vi "7-OCU Dave.vi"() -> ()   [LabVIEW 2010]
doc: "This VI contrains the Forebrain within the Olin Robot Architecture. It must be run first to load the appropriate mission definition files. It contains a finite state machine built around a tabbed Operator interface that will guide an operator through the startup, run shutdown mission sequence. After running it, run the Midbrain and Hindbrain VIS."
uses:
  7-OCU/TabEnum.ctl
  4-High Neurons/MDFArray.ctl
  4-High Neurons/MissionDefinitionFile.ctl
  6-OCU Neurons/6.1-Act.ctl
  6-OCU Neurons/MainIndicators.ctl
  4-High Neurons/Current GPS Data.ctl
  3-Midbrain/3.2-Where/_typedefs/3.2.1-VectorNav Data.ctl
  4-High Neurons/4.2-Where Sensor Typedef.ctl
  3-Midbrain/3.3-What/_typedefs/3.3.1-LIDAR Data Typedef.ctl
  4-High Neurons/4.3-What Sensor Typedef.ctl
  6-OCU Neurons/6.4-How Reporting Typedef.ctl
  6-OCU Neurons/6.1-UDP Saitek.ctl
panel:
  out "ignore me 2":bool
  out "ignore me":bool
  in  "MissionDefinition":T1={"Waypoint #"=2.0, "X (waypoint)"=0.0, "Y (waypoint)"=0.0, "Vel (desired)"=0.0, "Dwell Time"=0.0, "Behavior"=enum."OpenFieldTransit", "Expand1"=0.0, "Expand2"=0.0, "Expand3"=0.0}
  out "(xr,yr) A":cluster{"X":dbl, "Y":dbl}
  out "What?Midbrain":cluster{"T":dbl, "Range":dbl, "Bearing":dbl}[](array[cluster])
  out "How?Midbrain":cluster{"T":dbl, "Battery":dbl, "Temp":dbl}
  out "What?Forebrain":cluster{"T":dbl, "Range":dbl, "Bearing":dbl}[](array[cluster])
  out "How?Forebrain":cluster{"T":dbl, "Battery":dbl, "Temp":dbl}
  out "Where? Forebrain":T2
  out "WhereAmI? Clean":T2
  out "(xr,yr)":cluster{"X":dbl, "Y":dbl}
  out "How?ForebrainOut":cluster{"T":dbl, "Battery":dbl, "Temp":dbl}
  out "How?MidbrainMM":cluster{"T":dbl, "Battery":dbl, "Temp":dbl}
  out "WhereAmI?MidB":T2
  out "Where?Forebrain":T2
  out "WhatAroundMe?MidB":cluster{"T":dbl, "Range":dbl, "Bearing":dbl}[](array[cluster])
  in  "RunRobot":bool
  out "Robot Live":bool
  in  "E-Stop":bool
  in  "Main Tab Interface":T3
  out "StartMissionMap":picture
  out "BatteryState":dbl(slide) scale=20.0..24.0
  out "LIDARCheck":picture
  out "MissionTime S&S":dbl(knob) scale=0.0..10.0
  out "CollisionWarning":bool
  out "DebugLIDAR":picture
  in  "SubPosition":T4 {"xrobot" min=0.0 max=300.0; "yrobot" min=0.0 max=300.0; "heading" min=-7.0 max=7.0 step=0.01}
  in  "LIDARControl":T5
  out "LIDAR Data (r:pixel b:degrees)":cluster{"Range":dbl, "Bearing":dbl}[](array[cluster])
  in  "Stop DebugSENSE":bool
  out "MissionMap":picture
  out "MDF Out":T6
  out "initialized MDF":T6
  in  "MDFile":T1
  out "Way Point Index":i32
  out "InitialWaypoint":cluster{"X":i16, "Y":i16}
  in  "Pen Color":u32(colorbox)=15671808
  in  "Select Pen Attributes":T7={"Width"=1, "Style"=enum."Solid"}
  out "Draw??":bool
  out "ManualActCommand":dbl[](array[numeric])
  out "Hypo Out":cluster{"Motor1":i16, "Motor 2":i16}
  out "NeoActCom":dbl[](array[numeric])
  out "SteerAngle":dbl
  in  "Load From File":bool
  in  "Save to File":bool
  out "MDF":T6
  in  "Select Your Behavior":T8(ring)
  out "No. of Waypoints":i32
  in  "Exit Planning":bool
  out "MissionDefFile":picture
  in  "RobotSpeed_Leg":dbl(slide) min=0.0 max=4.0 step=0.01 scale=0.0..4.0
  out "BuildMDF":bool
  out "ManualModeDatums":T9 {"5.3.1 MissionTimeAuto" scale=0.0..10.0; "4.2-Where Am I? Sensor"."4.2.2- Current GPS Data"."Longitude (dd.mmmmmm)" format="%#.6g"; "4.2-Where Am I? Sensor"."4.2.2- Current GPS Data"."Lattitude (dd.mmmmmm)" format="%#.6g"}
  in  "AutoModeDatums":T16 {"6.1-Saitek Controller"."Right" scale=-32767.0..32767.0; "6.1-Saitek Controller"."Left" scale=-32767.0..32767.0; "6.1-Saitek Controller"."Yaw" scale=-32767.0..32767.0; "6.1-Saitek Controller"."Roll" scale=-32767.0..32767.0; "6.1-Saitek Controller"."Pitch" scale=-32767.0..32767.0}
  out "Indicators":T9 {"5.3.1 MissionTimeAuto" scale=0.0..10.0; "4.2-Where Am I? Sensor"."4.2.2- Current GPS Data"."Longitude (dd.mmmmmm)" format="%#.6g"; "4.2-Where Am I? Sensor"."4.2.2- Current GPS Data"."Lattitude (dd.mmmmmm)" format="%#.6g"}
  out "Ready":bool
  out "CollisionLight 2":bool
  # "To run\nrobot,\nclick\narrow\nabove\n\nTo shut \noff \nrobot,\nclick \nbutton\nbelow."
  # "Operation Directions\n\n1)Click on Startup&\nShutdown tab.\n2) Click on Run \nArrow on menubar.\nRun Forebrain,\nMidbrain and Hindbrain.\n3) Select a mssion \nmap file when asked.\n4) Check robot is \nfully operational on\nStartup tab.\n5) Debug with debug\ntabs as required.\n6) Select ManualMode\ntab and test drive \nrobot.\n7) Select PlanMission\ntab and set up \nmission.\n8) Go to AutoMode\ntab and run mission."
  # "Turns off drive\nmotors"
  # "To operate:\n1) Run Forebrain.vi\n2) Run Midbrain.vi\n3) Run Hindbrain.vi"
  # "Use this tab\nto explore\nLIDAR\ndata and \noperation"
  # "Set \nX=130\nY=100\nto put\nrobot\nin center of\nMission\nMap"
  # "Set\nNumberOfBeams\nSensorRange\nNoise\nto\nview\nsimulated\nsensor\ndata"
  # "Directions:\n1) Select Robot Behavior for each mission leg.\n2) Select Robot Speed for leg.\n3) Select Robot Depth for leg.\n4) Click on robots current location for first waypoint.\n5) Click on next waypoint. Repeat for full mission.\n6) MDF will store up to 20 waypoints."
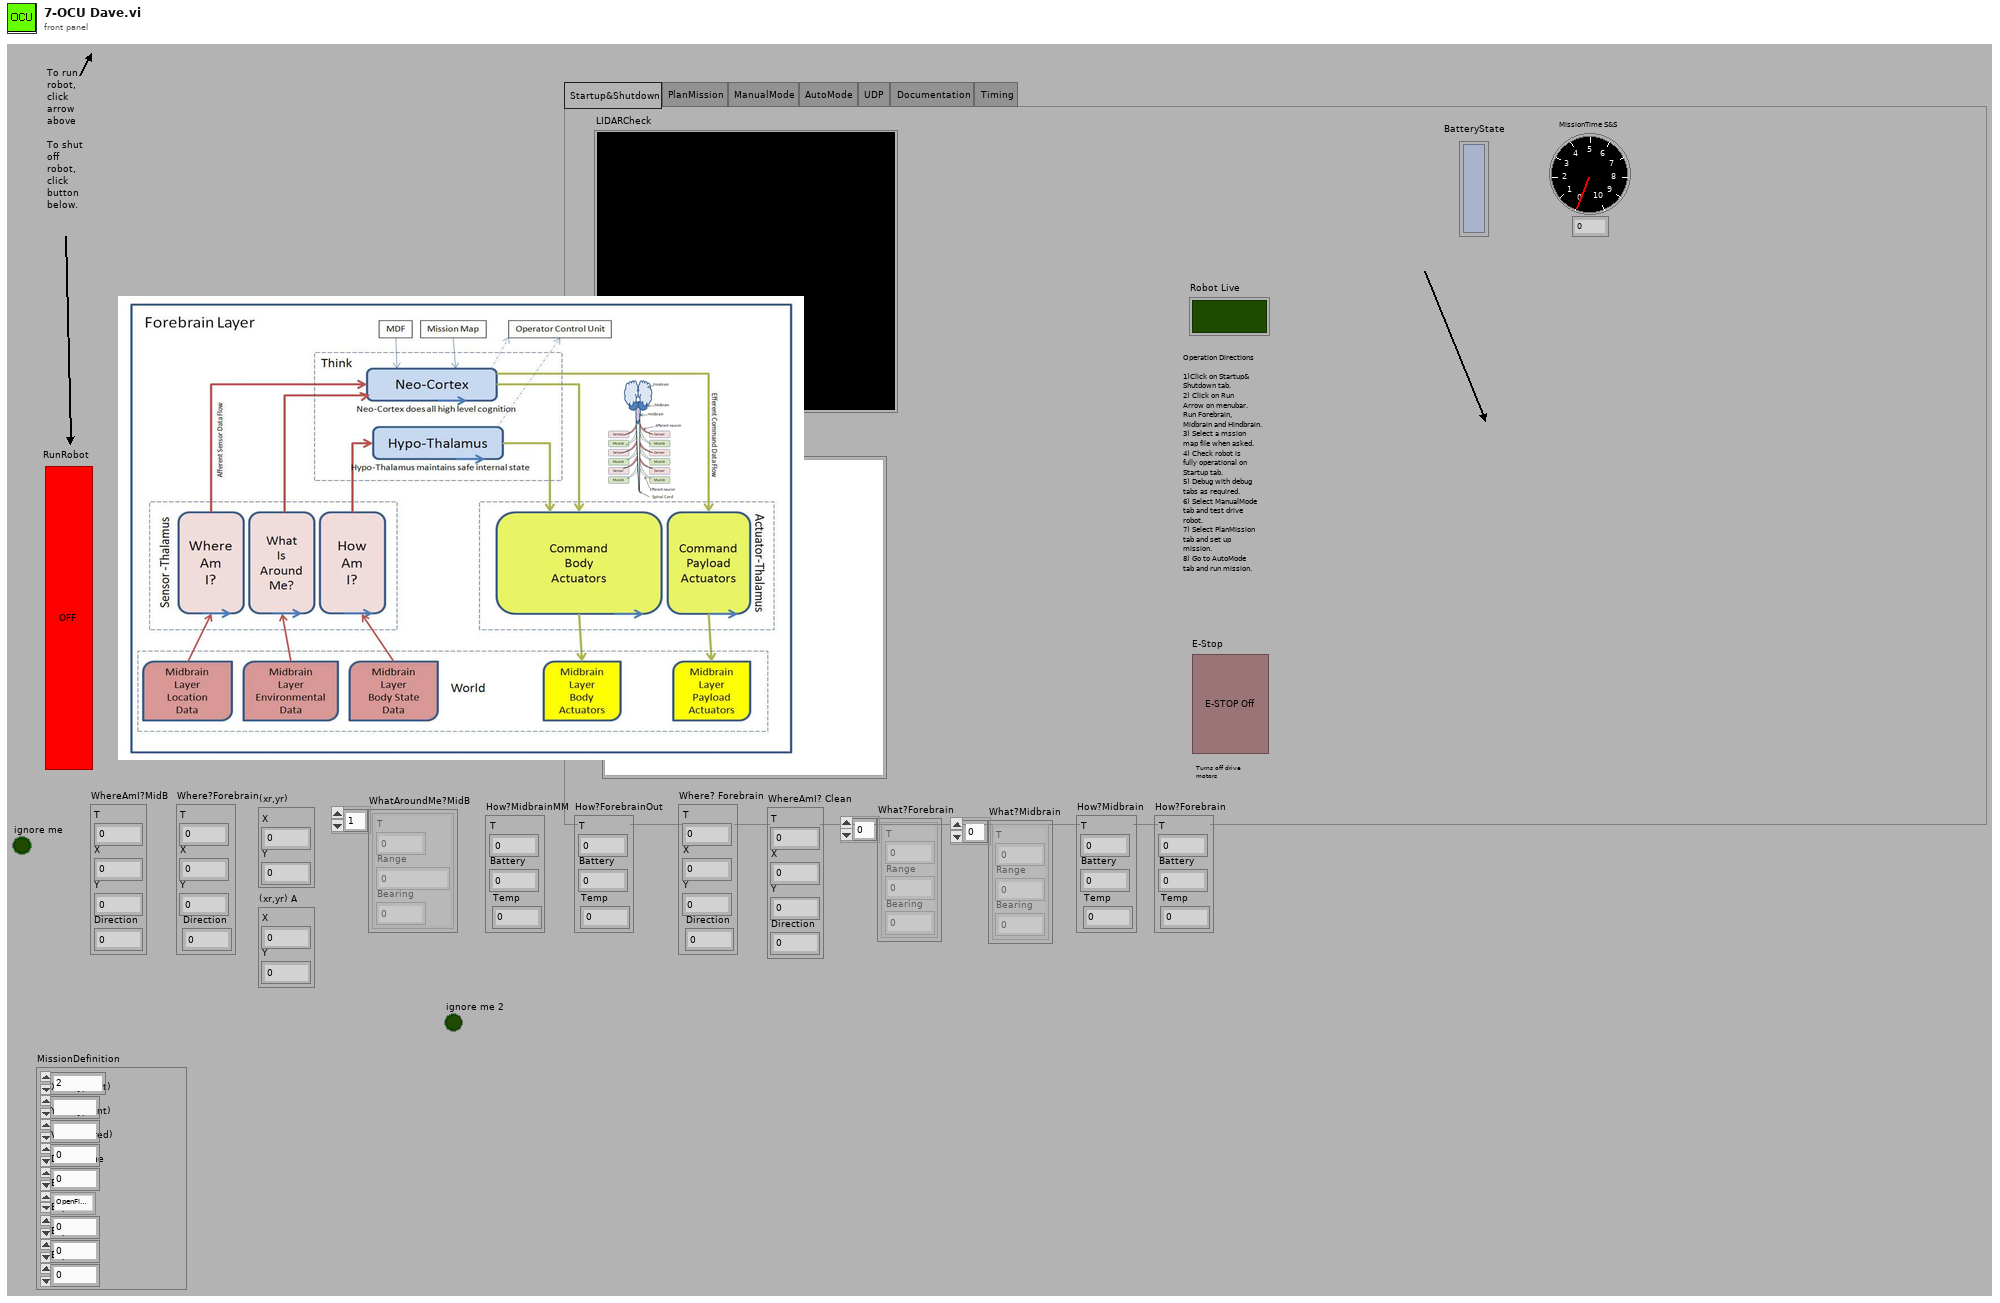
[diagram p1: front panel]
types:
  T1 = typedef "MissionDefinitionFile.ctl" = cluster{"Waypoint #":dbl, "X (waypoint)":ext, "Y (waypoint)":ext, "Vel (desired)":dbl, "Dwell Time":dbl, "Behavior":enum16{"OpenFieldTransit", "WallFollow", "LaneFollow", "ManualMode"}, "Expand1":dbl, "Expand2":dbl, "Expand3":dbl}
  T2 = cluster{"T":dbl, "X":dbl, "Y":dbl, "Direction":dbl}
  T3 = typedef "TabEnum.ctl" = enum32{"Startup&Shutdown", "PlanMission", "ManualMode", "AutoMode", "UDP", "Documentation", "Timing"}
  T4 = cluster{"xrobot":dbl, "yrobot":dbl, "heading":dbl}
  T5 = cluster{"NumberOfBeams":i32, "SensorRange":dbl, "Noise (0.1 to 1)":dbl}
  T6 = typedef "MDFArray.ctl" = T1[]
  T7 = cluster{"Width":u16, "Style":enum32{"Solid", "Dash", "Dot", "DashDot", "DashDotDot"}}
  T8 = enum16{"OpenFieldTransit", "WallFollow", "LaneFollow", "ManualMode"}
  T9 = typedef "MainIndicators.ctl" = cluster{"Where?":bool, "What?":bool, "4.2-Where Am I? Sensor":T10, "4.3-What's Around Me? Sensor":T13, "5.3.1 MissionTimeAuto":dbl, "5.4 Clean How Am I? Sensor":T15, "How?":bool}
  T10 = typedef "4.2-Where Sensor Typedef.ctl" = cluster{"4.2.2- Current GPS Data":T11, "4.2.1-VectorNav Data":T12, "4.2.1-VectorNav Status":string}
  T11 = typedef "Current GPS Data.ctl" = cluster{"Lattitude (dd.mmmmmm)":ext, "Longitude (dd.mmmmmm)":ext, "EST Time":timestamp}
  T12 = typedef "3.2.1-VectorNav Data.ctl" = cluster{"Yaw":dbl, "Pitch":dbl, "Roll":dbl}
  T13 = typedef "4.3-What Sensor Typedef.ctl" = cluster{"LIDAR Data":T14}
  T14 = typedef "3.3.1-LIDAR Data Typedef.ctl" = cluster{"Angle array":dbl[], "Magnitude array ":dbl[]}
  T15 = typedef "6.4-How Reporting Typedef.ctl" = cluster{"Motor Speed":i32, "Lidar Declination":i32, "Steering Angle":i32, "Battery Voltage":dbl, "Drive Encoder Cable Check":bool, "Lidar Drive Encoder Cable Check":bool, "Steer Encoder Cable Check":bool, "Lidar Pos Encoder Cable Check":bool, "Mod Buttons & Blinky Cable Check":bool, "Lidar Data Cable Check":bool, "Drive Motor Cable Check":bool, "Vector Nav Cable Check":bool, "Lidar Drive Cable Check":bool, "Steer Drive Cable Check":bool, "Reverse?":bool, "Steering Control Voltage":dbl, "Drive Control Voltage":dbl, "Lidar Control Voltage":dbl}
  T16 = typedef "6.1-Act.ctl" = cluster{"6.1-Saitek Controller":T17, "Manual Override":bool, "Shutdown":bool, "Reset":bool, "Begin":bool}
  T17 = typedef "6.1-UDP Saitek.ctl" = cluster{"Trig":bool, "2":bool, "3":bool, "4":bool, "5":bool, "6":bool, "7":bool, "8":bool, "9":bool, "10":bool, "11":bool, "Pitch":i32, "Ang":bool[], "Wheel":dbl, "Roll":i32, "Yaw":i32, "Left":i32, "Right":i32}
  T18 = enum32{"Startup&Shutdown", "DebugSENSE", "DebugTHINK", "DebugACT", "PlanMission", "ManualMode", "AutoMode", "Documentation"}
  T19 = cluster{"VelCom":dbl, "BehCom":enum16{"OpenFieldTransit", "WallFollow", "LaneFollow", "ManualMode"}}
  T20 = typedef "IMAQ Image.ctl" = refnum<image>
  T21 = typedef "imagedata.ctl" = cluster{"image type":i32, "image depth":i32, "image":u8[], "mask":u8[], "colors":u32[], "Rectangle":cluster{"left":i16, "top":i16, "right":i16, "bottom":i16}}
  T22 = typedef "LVMouseTypeDef.ctl" = cluster{"Mouse Position":cluster{"X":i32, "Y":i32}, "Mouse Modifiers":cluster{"Button Down":bool, "Shift Mod":bool, "Menu Mod":bool, "Option Mod":bool}}
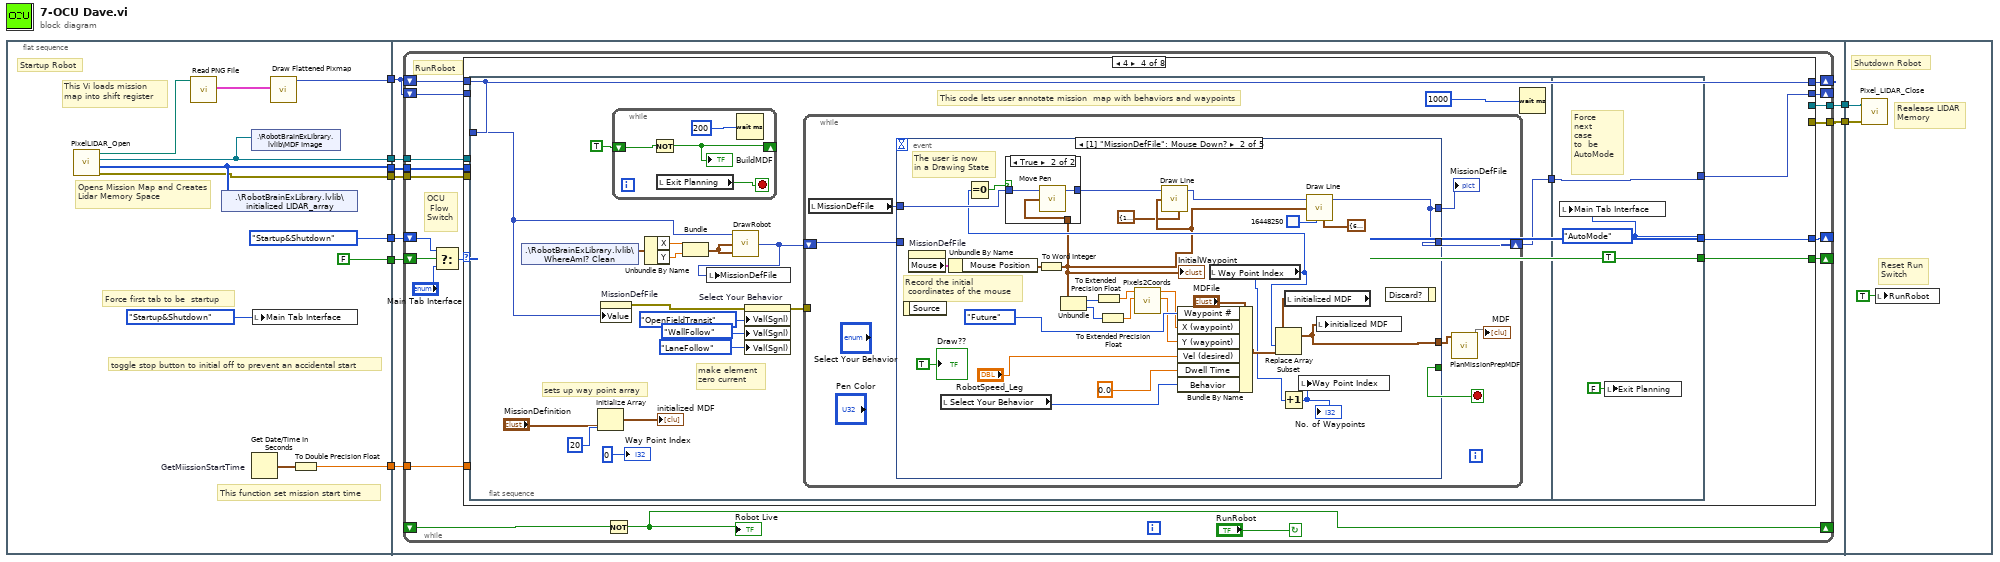
[diagram p0: block diagram]
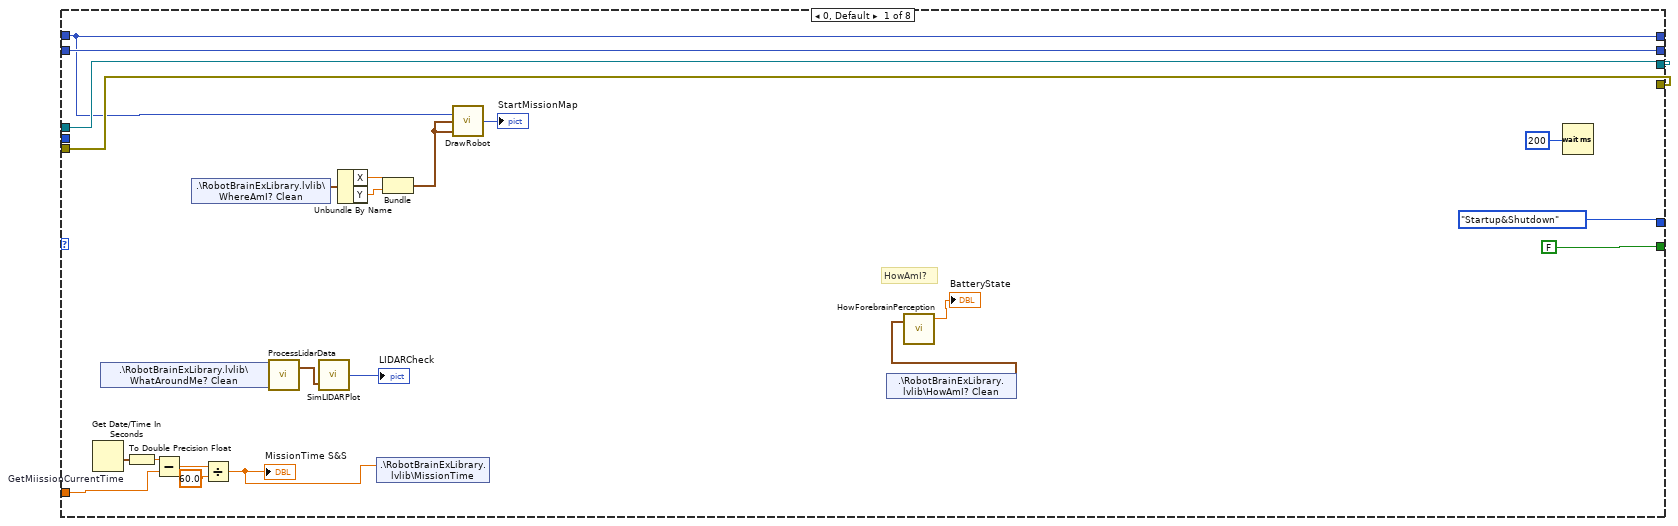
[diagram p2: hidden frame]
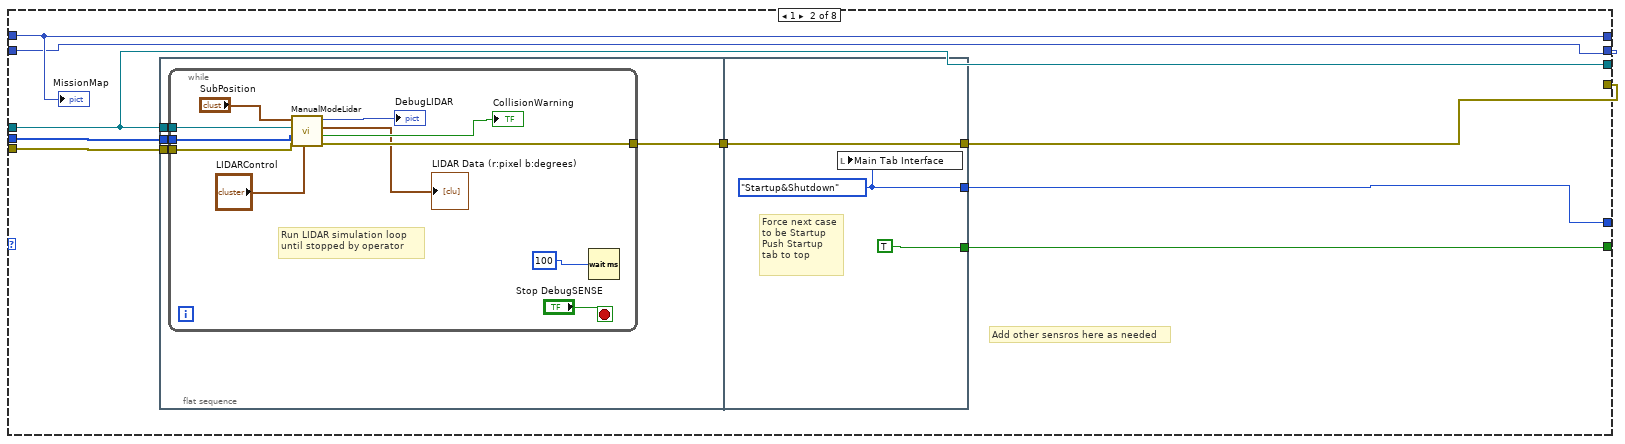
[diagram p3: hidden frame]
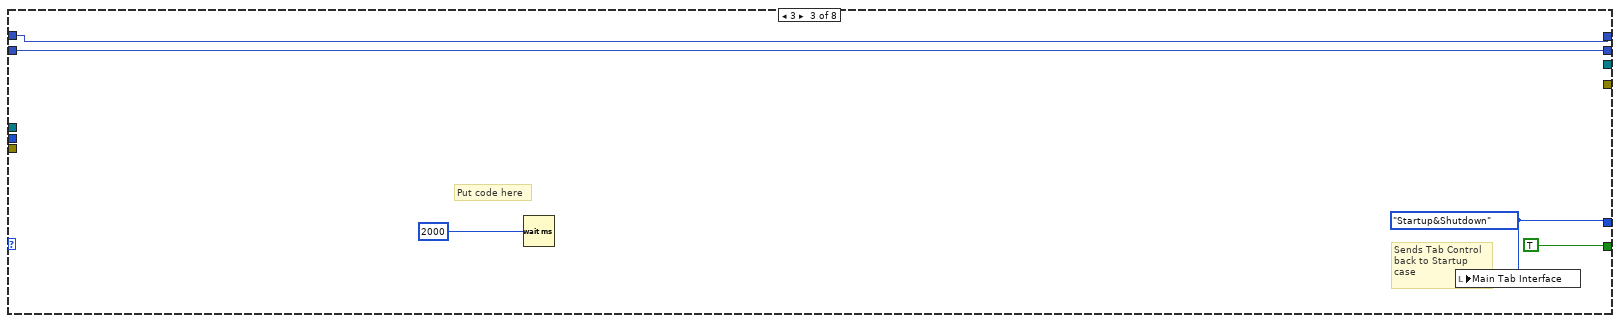
[diagram p4: hidden frame]
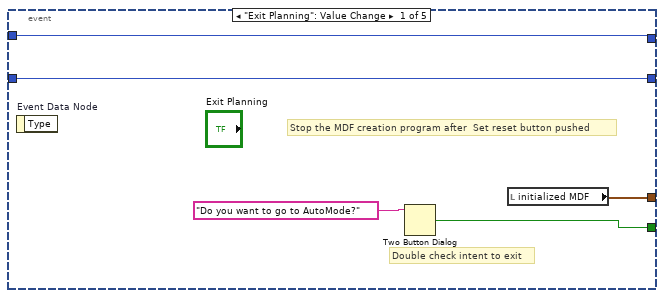
[diagram p5: hidden frame]
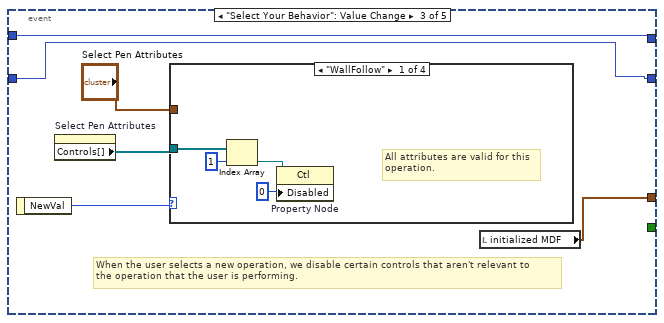
[diagram p7: hidden frame]
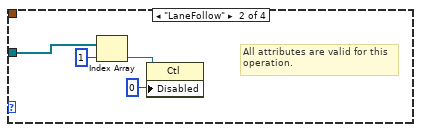
[diagram p8: hidden frame]
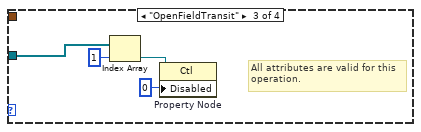
[diagram p9: hidden frame]
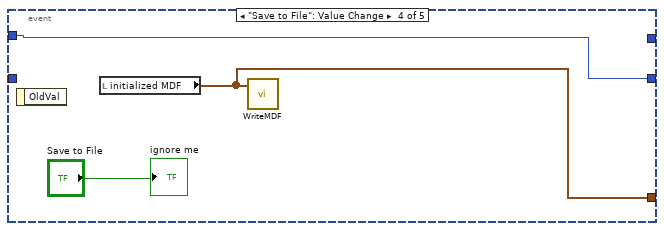
[diagram p11: hidden frame]
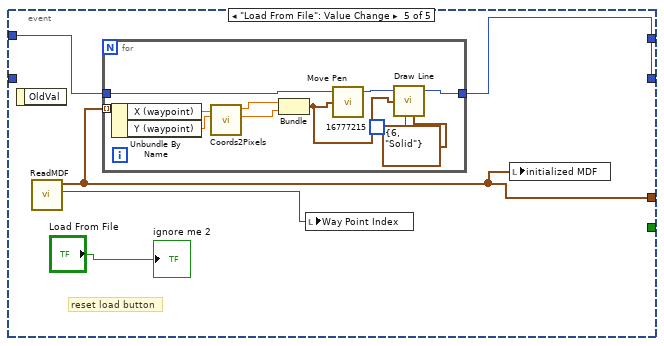
[diagram p12: hidden frame]
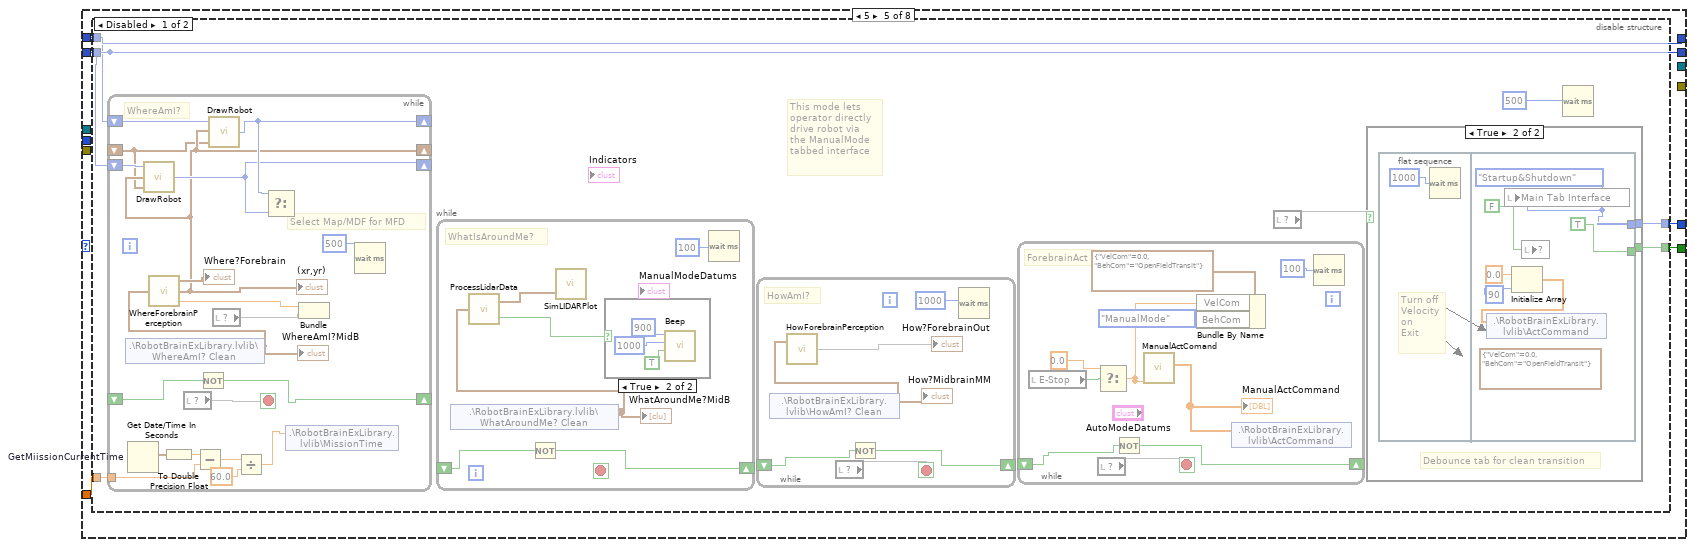
[diagram p13: hidden frame]
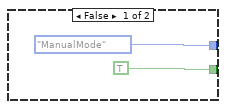
[diagram p15: hidden frame]
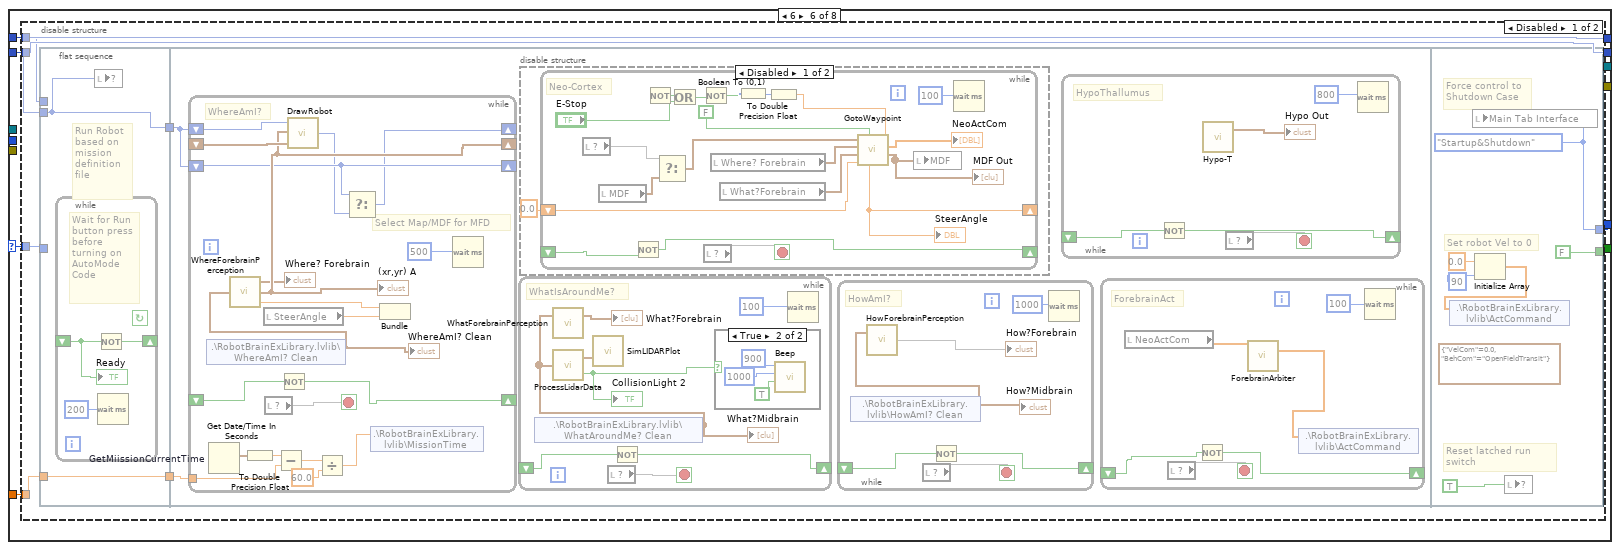
[diagram p17: hidden frame]
diagram:
  n1 = flat-sequence {
    tunnel: [w19] -> w9
    tunnel: [w17] -> w8
    tunnel: [w13] -> w7
    tunnel: [w15] -> w6
    tunnel: [w14] -> w5
    tunnel: [FALSE ("RunAutoMode")] -> w2
    tunnel: [T18."Startup&Shutdown" ("Tab")] -> w1
    tunnel: w9 -> [w29]
    tunnel: w8 -> [w28]
    tunnel: w7 -> [w27]
    tunnel: w6 -> [w26]
    tunnel: w5 -> [w25]
    tunnel: [w24] -> w4
    tunnel: [w23] -> w3
    tunnel: w2 -> [w22]
    tunnel: w1 -> [w21]
    tunnel: w4 -> [w405]
    tunnel: w3 -> [w404]
    frame #0 {
      # "Force first tab to be  startup"
      # "toggle stop button to initial off to prevent an accidental start"
      # "Opens Mission Map and Creates Lidar Memory Space"
      # "This function set mission start time"
      # "This Vi loads mission map into shift register"
      # "Startup Robot"
      n2 = call "PixelLIDAR_Open.vi"() -> ("error out"=w14:errorcluster, "initialized LIDAR\narray"=w15:i32[], "MDF Image"=w13:T20, "MissionMap"=w16:path)  [unwired: 2 in]
      n3 = call <vilib>:"Read PNG File.vi"("path to PNG file"=w16) -> ("image data"=w18:T21)  [unwired: 8 in, 2 out]
      n4 = shared-variable ".\\RobotBrainExLibrary.lvlib\\initialized LIDAR_array"(w15) -> ()  [unwired: 1 in, 1 out]
      n5 = shared-variable ".\\RobotBrainExLibrary.lvlib\\MDF Image"(w13) -> ()  [unwired: 1 in, 1 out]
      n6 = Get Date/Time In Seconds "GetMiissionStartTime"() -> (seconds since 1Jan1904=w20:timestamp)
      n7 = local write "Main Tab Interface"(T18."Startup&Shutdown" ("Tab")) -> ()
      n8 = call <vilib>:"Draw Flattened Pixmap.vi"("image data"=w18) -> ("new picture"=w17:picture)  [unwired: 8 in]
      n9 = To Double Precision Float(number=w20) -> (double precision float=w19:dbl)
    }
    frame #1 {
      n10 = while {
        shift-right: [w30] -> _
        shift-left: _ -> [w47]
        shift-right: [w46] -> _
        shift-left: w21 -> [w45]
        shift-right: [w42] -> _
        shift-left: w22 -> [w41]
        tunnel: w29 -> [w40]
        shift-right: [w38] -> _
        shift-left: w28 -> [w39]
        shift-right: [w36] -> _
        shift-left: w28 -> [w37]
        tunnel: w27 -> [w35]
        tunnel: w26 -> [w34]
        tunnel: w25 -> [w33]
        tunnel: [w32] -> w24
        tunnel: [w31] -> w23
        stop <- "RunRobot" continue-if-true
        # "RunRobot"
        # "OCU\n Flow\nSwitch"
        n11 = Select(t=w45, s=w41, f="Main Tab Interface") -> (s? t:f=w43:u32)
        n12 = case shown="4" w43 {
          selector: w43 -> [_ _ _ _ _ w296 _ _]
          tunnel: [T18."Startup&Shutdown" ("Tab") w75 w101 w108 w219 w297 T18."Startup&Shutdown" ("Tab") w402] -> w46
          tunnel: [FALSE ("s") w74 TRUE ("s") w107 w220 w295 FALSE ("s") TRUE ("s")] -> w42
          tunnel: w40 -> [w64 _ _ _ w218 w294 _ _]
          tunnel: w39 -> [w56 w77 w100 w104 w216 w292 w395 w400]
          tunnel: [w56 w77 w100 w104 w216 w292 w395 w400] -> w38
          tunnel: w37 -> [w63 w72 w99 _ w217 w293 w394 w399]
          tunnel: [w63 w72 w99 w105 w217 w293 w394 w399] -> w36
          tunnel: w35 -> [w62 w73 _ _ _ _ _ _]
          tunnel: w34 -> [_ w80 _ _ _ _ _ _]
          tunnel: w33 -> [w61 w79 _ _ _ _ _ _]
          tunnel: [w62 w73 _ _ _ _ _ _] -> w32
          tunnel: [w61 w78 _ _ _ _ _ _] -> w31
          frame 0, Default {
            # "HowAmI?"
            n13 = Get Date/Time In Seconds "GetMiissionCurrentTime"() -> (seconds since 1Jan1904=w68:timestamp)
            n14 = shared-variable ".\\RobotBrainExLibrary.lvlib\\WhatAroundMe? Clean"() -> (w57:cluster{"T":dbl, "Range":dbl, "Bearing":dbl}[])  [unwired: 1 in, 1 out]
            n15 = To Double Precision Float(number=w68) -> (double precision float=w67:dbl)
            n16 = Subtract(x=w67, y=w64) -> (x-y=w66:dbl)
            n17 = shared-variable ".\\RobotBrainExLibrary.lvlib\\WhereAmI? Clean"() -> (w52:T2)  [unwired: 1 in, 1 out]
            n18 = Divide(x=w66, y=60.0) -> (x/y=w60:dbl)
            "MissionTime S&S" <- w60
            n19 = call "ProcessLidarData.vi"("WhatAroundMe?MM"=w57) -> ("data array [mag, phase (deg)]"=w58:cluster{"magnitude":dbl, "phase":dbl}[])  [unwired: 1 out]
            n20 = call "SimLIDARPlot.vi"("data array [mag, phase (deg)]"=w58) -> ("SONAR"=→"LIDARCheck":picture)  [unwired: 1 in]
            n21 = Unbundle By Name(w52) -> ("X"=w51:dbl, "Y"=w50:dbl)
            n22 = shared-variable ".\\RobotBrainExLibrary.lvlib\\MissionTime"(w60) -> ()  [unwired: 1 in, 1 out]
            n23 = Bundle("X"=w51, "Y"=w50) -> (w49:cluster{"X":dbl, "Y":dbl})  [unwired: 1 in]
            n24 = call "DrawRobot.vi"("(xr,yr) old"=w49, "(xr,yr) new"=w49, "2D Picture"=w56) -> ("new picture"=→"StartMissionMap":picture)
            n25 = shared-variable ".\\RobotBrainExLibrary.lvlib\\HowAmI? Clean"() -> (w54:cluster{"T":dbl, "Battery":dbl, "Temp":dbl})  [unwired: 1 in, 1 out]
            n26 = call "HowForebrainPerception.vi"("How?MidbrainIn"=w54) -> ("BatteryGauge"=→"BatteryState":dbl)  [unwired: 3 in]
            n27 = Wait (ms)(milliseconds to wait=u32 200) -> ()  [unwired: 1 out]
          }
          frame 1 {
            # "Add other sensros here as needed"
            n28 = flat-sequence {
              tunnel: w80 -> [w84]
              tunnel: w79 -> [w83]
              tunnel: w73 -> [w82]
              tunnel: [w81] -> w76
              tunnel: [w98] -> w78
              tunnel: w76 -> [w98]
              tunnel: [w97] -> w75
              tunnel: [TRUE ("s")] -> w74
              frame #0 {
                n29 = while {
                  tunnel: w84 -> [w95]
                  tunnel: w83 -> [w94]
                  tunnel: w82 -> [w93]
                  tunnel: [w92] -> w81
                  stop <- "Stop DebugSENSE" stop-if-true
                  # "Run LIDAR simulation loop\nuntil stopped by operator"
                  n30 = call "ManualModeLidar.vi"("LIDARControl"="LIDARControl", "error in"=w94, "initialized \nsonar ray\narray"=w95, "MDF Image"=w93, "SubPosition"="SubPosition") -> ("error out"=w92:errorcluster, "Collision\nWarning"=→"CollisionWarning":bool, "LIDAR Data (r:pixel b:degrees)"=→"LIDAR Data (r:pixel b:degrees)":cluster{"Range":dbl, "Bearing":dbl}[], "LIDAR"=→"DebugLIDAR":picture)  [unwired: 1 in]
                  n31 = Wait (ms)(milliseconds to wait=u32 100) -> ()  [unwired: 1 out]
                }
              }
              frame #1 {
                w97 = T18."Startup&Shutdown" ("Tab")
                # "Force next case\nto be Startup\nPush Startup\ntab to top"
                n32 = local write "Main Tab Interface"(w97) -> ()
              }
            }
            "MissionMap" <- w77
          }
          frame 3 {
            w101 = T18."Startup&Shutdown" ("Tab")
            # "Put code here"
            # "Sends Tab Control\nback to Startup\ncase"
            n33 = Wait (ms)(milliseconds to wait=u32 2000) -> ()  [unwired: 1 out]
            n34 = local write "Main Tab Interface"(w101) -> ()
          }
          frame 4 {
            n35 = flat-sequence {
              tunnel: [w125] -> w106
              tunnel: w104 -> [w110]
              tunnel: [w214] -> w108
              tunnel: [TRUE ("s")] -> w107
              tunnel: w106 -> [w213]
              tunnel: [w213] -> w105
              frame #0 {
                # "make element \nzero current"
                # "sets up way point array"
                # "This code lets user annotate mission  map with behaviors and waypoints"
                n36 = shared-variable ".\\RobotBrainExLibrary.lvlib\\WhereAmI? Clean"() -> (w114:T2)  [unwired: 1 in, 1 out]
                n37 = Initialize Array ("Initialize WaypointArray")("MissionDefinition", 20 ("dimension size")) -> (→"initialized MDF":T1[])
                n38 = property on="MissionDefFile" class="Pict"("Value"=w110) -> (error out=w123:errorcluster)  [unwired: 2 in, 1 out]
                n39 = while {
                  shift-right: [w129] -> _
                  shift-left: TRUE -> [w130]
                  stop <- w128 stop-if-true
                  n40 = Not(x=w130) -> (.not. x?=w129:bool)
                  "BuildMDF" <- w129
                  n41 = local read "Exit Planning"() -> (w128:bool)
                  n42 = Wait (ms)(milliseconds to wait=u32 200) -> ()  [unwired: 1 out]
                }
                n43 = Unbundle By Name(w114) -> ("X"=w113:dbl, "Y"=w112:dbl)
                n44 = Bundle("X"=w113, "Y"=w112) -> (w111:cluster{"X":dbl, "Y":dbl})  [unwired: 1 in]
                n45 = call "DrawRobot.vi"("(xr,yr) old"=w111, "(xr,yr) new"=w111, "2D Picture"=w110) -> ("new picture"=w109:picture)
                n46 = local write "MissionDefFile"(w109) -> ()
                n47 = property on="Select Your Behavior" class="Enum (strict)"(error in=w123, "Val(Sgnl)"=T8."OpenFieldTransit" ("Select Your Behavior"), "Val(Sgnl)"=T8."WallFollow" ("Value (Signaling)"), "Val(Sgnl)"=T8."LaneFollow" ("Select Your Behavior")) -> (error out=w124:errorcluster)  [unwired: 1 in, 1 out]
                n48 = while {
                  shift-right: [w136] -> w125
                  shift-left: w109 -> [w137]
                  tunnel: w124 -> [_]
                  stop <- w135 stop-if-true
                  n49 = local read "MissionDefFile"() -> (w134:picture)
                  n50 = event shown="[1] \"MissionDefFile\": Mouse Down?" {
                    selector: _ -> [_ _ _ _ _]
                    dyn-events: _ -> [_ _ _ _ _]
                    timeout: _ -> [_ _ _ _ _]
                    tunnel: [w140 w153 w175 w194 w196] -> w136
                    tunnel: w137 -> [w140 _ w175 _ _]
                    tunnel: [w141 _ _ _ _] -> w135
                    tunnel: [w139 w167 w177 w195 w198] -> w131
                    tunnel: w134 -> [w138 w154 w176 w194 w197]
                    tunnel: [w138 w153 w176 _ _] -> w133
                    event "Exit Planning": Value Change {
                      # "Double check intent to exit"
                      # "Stop the MDF creation program after  Set reset button pushed"
                      n51 = event-data "Event Data Node"() -> ()  [unwired: 1 in, 1 out]
                      n52 = Two Button Dialog(message="Do you want to go to AutoMode?") -> (T button?=w141:bool)  [unwired: 2 in]
                      n53 = local read "initialized MDF"() -> (w139:T6)
                    }
                    event "MissionDefFile": Mouse Down? {
                      # "Record the initial\n coordinates of the mouse"
                      # "The user is now\nin a Drawing State"
                      n54 = event-data() -> ()  [unwired: 1 in, 1 out]
                      n55 = property on="MissionDefFile" class="Pict"() -> ("Mouse"=w170:T22)  [unwired: 2 in, 2 out]
                      n56 = local read "Select Your Behavior"() -> (w161:T8)
                      n57 = Unbundle By Name(w170) -> ("Mouse Position"=w168:cluster{"X":i32, "Y":i32})
                      n58 = To Word Integer(number=w168) -> (16bit integer=w144:cluster{"X":i16, "Y":i16})
                      "InitialWaypoint" <- w144
                      n59 = Unbundle(w144) -> ("X"=w163:i16, "Y"=w162:i16)
                      n60 = To Extended Precision Float(1:w163) -> (0:w151:ext)
                      n61 = To Extended Precision Float(1:w162) -> (0:w150:ext)
                      n62 = call "Pixels2Coords.vi"("Y (pixels)"=w150, "X (pixels)"=w151) -> ("Latitude"=w148:ext, "Longtitude"=w149:ext)  [unwired: 8 in]
                      n63 = Bundle By Name(cluster="MDFile", "Waypoint #"=enum16{"Past", "Current", "Future"}."Future" ("Status"), "X (waypoint)"=w149, "Y (waypoint)"=w148, "Vel (desired)"="RobotSpeed_Leg", "Dwell Time"=0.0, "Behavior"=w161) -> (w164:T1)
                      n64 = local read "Way Point Index"() -> (w147:i32)
                      n65 = Equal To 0?(x=w147) -> (x = 0?=w146:bool)
                      n66 = case shown="True" w146 {
                        tunnel: [w171 w174] -> w157
                        tunnel: w144 -> [_ w173]
                        tunnel: w154 -> [w171 w172]
                        frame False {
                        }
                        frame True {
                          n67 = call <vilib>:"Move Pen.vi"("new position"=w173, "picture"=w172) -> ("new picture"=w174:picture)  [unwired: 3 in]
                        }
                      }
                      n68 = call <vilib>:"Draw Line.vi"("picture"=w157, "end point"=w144, "pen"=T7 {"Width"=1, "Style"=enum."Dot"}) -> ("new picture"=w145:picture)  [unwired: 6 in]
                      n69 = Increment(x=w147) -> (x+1=w169:i32)
                      "No. of Waypoints" <- w169
                      n70 = local read "initialized MDF"() -> (w166:T6)
                      n71 = Replace Array Subset(array=w166, new element=w164, index=w147) -> (w167:T6)
                      n72 = local write "Way Point Index"(w169) -> ()
                      n73 = call <vilib>:"Draw Line.vi"("picture"=w145, "end point"=w144, "color(black)"=u32 16448250, "pen"=T7 {"Width"=6, "Style"=enum."Solid"}) -> ("new picture"=w153:picture)  [unwired: 5 in]
                      n74 = local write "initialized MDF"(w167) -> ()
                      n75 = event-data() -> ()  [unwired: 2 in, 1 out]
                      "Draw??" <- TRUE ("Draw??")
                    }
                    event "Select Your Behavior": Value Change {
                      # "When the user selects a new operation, we disable certain controls that aren't relevant to\nthe operation that the user is performing."
                      n76 = event-data() -> ("NewVal"=w180:T8)  [unwired: 1 in]
                      n77 = property on="Select Pen Attributes" class="Clust (strict)"() -> ("Controls[]"=w179:refnum<vi>[])  [unwired: 2 in, 2 out]
                      n78 = case shown="\"WallFollow\"" w180 {
                        tunnel: w179 -> [w184 w185 w189 _]
                        tunnel: "Select Pen Attributes" -> [_ _ _ _]
                        frame "WallFollow" {
                          # "All attributes are valid for this\noperation."
                          n79 = Index Array "Index Array"(array=w184, index=1) -> (element=w182:refnum<vi>)
                          n80 = property on="Property Node" class="Ctl"(reference=w182, "Disabled"=u8 0) -> ()  [unwired: 1 in, 2 out]
                        }
                        frame "LaneFollow" {
                          # "All attributes are valid for this\noperation."
                          n81 = Index Array(array=w185, index=1) -> (element=w187:refnum<vi>)
                          n82 = property class="Ctl"(reference=w187, "Disabled"=u8 0) -> ()  [unwired: 1 in, 2 out]
                        }
                        frame "OpenFieldTransit" {
                          # "All attributes are valid for this\noperation."
                          n83 = Index Array "Index Array"(array=w189, index=1) -> (element=w191:refnum<vi>)
                          n84 = property on="Property Node" class="Ctl"(reference=w191, "Disabled"=u8 0) -> ()  [unwired: 1 in, 2 out]
                        }
                        frame "ManualMode" {
                        }
                      }
                      n85 = local read "initialized MDF"() -> (w177:T6)
                    }
                    event "Save to File": Value Change {
                      n86 = event-data() -> ()  [unwired: 1 in, 1 out]
                      n87 = local read "initialized MDF"() -> (w195:T6)
                      n88 = call "WriteMDF.vi"(11:w195) -> ()  [unwired: 11 in]
                      "ignore me" <- "Save to File"
                    }
                    event "Load From File": Value Change {
                      # "reset load button"
                      n89 = event-data() -> ()  [unwired: 1 in, 1 out]
                      n90 = call "ReadMDF.vi"() -> ("Number of Waypoints Read"=w199:i32, "MDF Array out"=w198:T6)  [unwired: 10 in]
                      n91 = for {
                        tunnel: w198 -> [w211] mode=indexing
                        tunnel: w197 -> [w210]
                        tunnel: [w208] -> w196
                        n92 = Unbundle By Name(w211) -> ("X (waypoint)"=w204:ext, "Y (waypoint)"=w203:ext)
                        n93 = call "Coords2Pixels.vi"("Latitude"=w203, "Longitude"=w204) -> ("Y"=w201:ext, "X"=w202:ext)  [unwired: 8 in]
                        n94 = Bundle("X"=w202, "Y"=w201) -> (w207:cluster{"X":ext, "Y":ext})  [unwired: 1 in]
                        n95 = call <vilib>:"Move Pen.vi"("new position"=w207, "picture"=w210) -> ("new picture"=w209:picture)  [unwired: 3 in]
                        n96 = call <vilib>:"Draw Line.vi"("picture"=w209, "end point"=w207, "color(black)"=u32 16777215, "pen"=T7 {"Width"=6, "Style"=enum."Solid"}) -> ("new picture"=w208:picture)  [unwired: 5 in]
                      }
                      n97 = local write "Way Point Index"(w199) -> ()
                      n98 = local write "initialized MDF"(w198) -> ()
                      "ignore me 2" <- "Load From File"
                    }
                  }
                  "MissionDefFile" <- w133
                  n99 = call "PlanMissionPrepMDF.vi"(11:w131) -> (3:→"MDF")  [unwired: 9 in, 1 out]
                }
                n100 = Wait (ms)(milliseconds to wait=u32 1000) -> ()  [unwired: 1 out]
                "Way Point Index" <- 0 ("Boundary Point Index")
              }
              frame #1 {
                w214 = T18."AutoMode" ("Tab")
                # "Force \nnext \ncase\nto  be\nAutoMode"
                n101 = local write "Main Tab Interface"(w214) -> ()
                n102 = local write "Exit Planning"(FALSE ("Exit Planning")) -> ()
              }
            }
          }
          frame 5 {
            n103 = disable-structure shown="Disabled" {
              disable-tunnel: [w226 _] -> w220
              disable-tunnel: [w225 _] -> w219
              disable-tunnel: w218 -> [w223 _]
              disable-tunnel: w217 -> [w222 _]
              disable-tunnel: w216 -> [w221 _]
              frame Disabled {
                # "This mode lets \noperator directly\ndrive robot via\nthe ManualMode\ntabbed interface"
                n104 = while {
                  shift-right: [w250] -> _
                  shift-left: _ -> [w249]
                  tunnel: w223 -> [w242]
                  shift-right: [w232] -> _
                  shift-left: w221 -> [w235]
                  shift-right: [w229] -> _
                  shift-left: _ -> [w228]
                  shift-right: [w230] -> _
                  shift-left: w222 -> [w231]
                  stop <- w248 stop-if-true
                  # "Select Map/MDF for MFD"
                  # "WhereAmI?"
                  n105 = shared-variable ".\\RobotBrainExLibrary.lvlib\\WhereAmI? Clean"() -> (w241:T2)  [unwired: 1 in, 1 out]
                  "WhereAmI?MidB" <- w241
                  n106 = Get Date/Time In Seconds "GetMiissionCurrentTime"() -> (seconds since 1Jan1904=w243:timestamp)
                  n107 = call "WhereForebrainPerception.vi"("Where? Midbrain"=w241) -> ("SimPitchRoll"=w240:dbl, "Where? Forebrain"=→"Where?Forebrain":T2, "(xr,yr)"=w229:cluster{"X":dbl, "Y":dbl}, "Direction"=w239:dbl)  [unwired: 3 in]
                  "(xr,yr)" <- w229
                  n108 = call "DrawRobot.vi"("(xr,yr) old"=w228, "(xr,yr) new"=w229, "2D Picture"=w231) -> ("new picture"=w230:picture)
                  n109 = To Double Precision Float(number=w243) -> (double precision float=w244:dbl)
                  n110 = local read item#-1() -> (w248)
                  n111 = Subtract(x=w244, y=w242) -> (x-y=w245:dbl)
                  n112 = Not(x=w249) -> (.not. x?=w250:bool)
                  n113 = call "DrawRobot.vi"("(xr,yr) old"=w228, "(xr,yr) new"=w229, "2D Picture"=w235) -> ("new picture"=w232:picture)
                  n114 = local read item#-1() -> (w237)
                  n115 = Divide(x=w245, y=60.0) -> (x/y=w247:dbl)
                  n116 = Select(t=w232, f=w230) -> (s=w233:bool, s? t:f=w234:picture)
                  n117 = shared-variable ".\\RobotBrainExLibrary.lvlib\\MissionTime"(w247) -> ()  [unwired: 1 in, 1 out]
                  n118 = Bundle("Direction"=w239, w237) -> (w238:cluster{"Direction":dbl, void})  [unwired: 1 in]
                  n119 = Wait (ms)(milliseconds to wait=u32 500) -> ()  [unwired: 1 out]
                }
                n120 = while {
                  shift-right: [w257] -> _
                  shift-left: _ -> [w258]
                  stop <- w256 stop-if-true
                  # "WhatIsAroundMe?"
                  n121 = shared-variable ".\\RobotBrainExLibrary.lvlib\\WhatAroundMe? Clean"() -> (w253:cluster{"T":dbl, "Range":dbl, "Bearing":dbl}[])  [unwired: 1 in, 1 out]
                  "WhatAroundMe?MidB" <- w253
                  n122 = call "ProcessLidarData.vi"("WhatAroundMe?MM"=w253) -> ("Collision"=w252:bool, "data array [mag, phase (deg)]"=w254:cluster{"magnitude":dbl, "phase":dbl}[])
                  n123 = Not(x=w258) -> (.not. x?=w257:bool)
                  n124 = call "SimLIDARPlot.vi"("data array [mag, phase (deg)]"=w254) -> ("SONAR"=w255:picture)  [unwired: 1 in]
                  n125 = case shown="True" w252 {
                    frame False {
                      # "No \nBeep"
                    }
                    frame True {
                      n126 = call <vilib>:"Beep.vi"("use system alert? (T)"=TRUE, "duration (msec)"=u32 1000, "frequency (Hz)"=u32 900) -> ()  [unwired: 9 in]
                    }
                  }
                  n127 = Wait (ms)(milliseconds to wait=u32 100) -> ()  [unwired: 1 out]
                }
                n128 = while {
                  shift-right: [w279] -> _
                  shift-left: _ -> [w278]
                  stop <- w275 stop-if-true
                  # "HowAmI?"
                  n129 = shared-variable ".\\RobotBrainExLibrary.lvlib\\HowAmI? Clean"() -> (w277:cluster{"T":dbl, "Battery":dbl, "Temp":dbl})  [unwired: 1 in, 1 out]
                  "How?MidbrainMM" <- w277
                  n130 = call "HowForebrainPerception.vi"("How?MidbrainIn"=w277) -> (3:→"How?ForebrainOut")  [unwired: 2 in, 1 out]
                  n131 = local read item#-1() -> (w275)
                  n132 = Not(x=w278) -> (.not. x?=w279:bool)
                  n133 = Wait (ms)(milliseconds to wait=u32 1000) -> ()  [unwired: 1 out]
                }
                n134 = while {
                  shift-right: [w273] -> _
                  shift-left: _ -> [w272]
                  stop <- w270 stop-if-true
                  # "ForebrainAct"
                  n135 = local read "E-Stop"() -> (w264:bool)
                  n136 = Select(t=0.0, s=w264) -> (f=w265:dbl, s? t:f=w266:dbl)
                  n137 = local read item#-1() -> (w270)
                  n138 = Not(x=w272) -> (.not. x?=w273:bool)
                  n139 = call "ManualActComand.vi"("Speed"=w266) -> ("ManualActCommand"=w271:dbl[], "SteeringAngle"=w269:dbl)  [unwired: 9 in]
                  "ManualActCommand" <- w271
                  n140 = Bundle By Name(cluster=T19 {"VelCom"=0.0, "BehCom"=enum."OpenFieldTransit"} ("ForebrainCom"), "VelCom"=w266, "BehCom"=T8."ManualMode") -> ()  [unwired: 1 out]
                  n141 = shared-variable ".\\RobotBrainExLibrary.lvlib\\ActCommand"(w271) -> ()  [unwired: 1 in, 1 out]
                  n142 = Wait (ms)(milliseconds to wait=u32 100) -> ()  [unwired: 1 out]
                }
                n143 = local read item#-1() -> (w224)
                n144 = case shown="True" w224 {
                  tunnel: [TRUE ("s") w283] -> w226
                  tunnel: [T18."ManualMode" ("Tab") w284] -> w225
                  frame False {
                  }
                  frame True {
                    # "Debounce tab for clean transition"
                    n145 = flat-sequence {
                      tunnel: [w290] -> w284
                      tunnel: [TRUE ("s")] -> w283
                      frame #0 {
                        # "Turn off\nVelocity\non \nExit"
                        n146 = Wait (ms)(milliseconds to wait=u32 1000) -> ()  [unwired: 1 out]
                      }
                      frame #1 {
                        (unwired) T19 {"VelCom"=0.0, "BehCom"=enum."OpenFieldTransit"} ("ForebrainCom")
                        w290 = T18."Startup&Shutdown" ("Tab")
                        n147 = local write "Main Tab Interface"(w290) -> ()
                        n148 = Initialize Array(0.0 ("element"), 90 ("dimension size")) -> (w288:dbl[])
                        n149 = shared-variable ".\\RobotBrainExLibrary.lvlib\\ActCommand"(w288) -> ()  [unwired: 1 in, 1 out]
                        n150 = local write item#-1(FALSE ("ManualModeStop")) -> ()
                      }
                    }
                  }
                }
                n151 = Wait (ms)(milliseconds to wait=u32 500) -> ()  [unwired: 1 out]
              }
              frame Enabled {
              }
            }
          }
          frame 6 {
            n152 = disable-structure shown="Disabled" {
              disable-tunnel: [w303 _] -> w297
              disable-tunnel: w296 -> [w302 _]
              disable-tunnel: [w301 _] -> w295
              disable-tunnel: w294 -> [w300 _]
              disable-tunnel: w293 -> [w299 _]
              disable-tunnel: w292 -> [w298 _]
              frame Disabled {
                n153 = flat-sequence {
                  tunnel: w302 -> [_]
                  tunnel: [w307] -> w305
                  tunnel: w300 -> [w307]
                  tunnel: w299 -> [w306]
                  tunnel: [w306] -> w304
                  tunnel: w298 -> [_]
                  tunnel: w305 -> [w312]
                  tunnel: w304 -> [w311]
                  tunnel: [w392] -> w303
                  tunnel: [FALSE ("s")] -> w301
                  frame #0 {
                    # "Run Robot\nbased on\nmission\ndefinition\nfile"
                    n154 = while {
                      shift-right: [w310] -> _
                      shift-left: _ -> [w309]
                      stop <- _ continue-if-true
                      # "Wait for Run\nbutton press\nbefore\nturning on\nAutoMode\nCode"
                      n155 = Not(x=w309) -> (.not. x?=w310:bool)
                      n156 = Wait (ms)(milliseconds to wait=u32 200) -> ()  [unwired: 1 out]
                      "Ready" <- w309
                    }
                    n157 = local write item#-1(w306) -> ()
                  }
                  frame #1 {
                    n158 = while {
                      shift-right: [w386] -> _
                      shift-left: _ -> [w373]
                      tunnel: w312 -> [w381]
                      shift-right: [w365] -> _
                      shift-left: w311 -> [w368]
                      shift-right: [w378] -> _
                      shift-left: _ -> [w379]
                      shift-right: [w367] -> _
                      shift-left: w311 -> [w367]
                      stop <- w372 stop-if-true
                      # "Select Map/MDF for MFD"
                      # "WhereAmI?"
                      n159 = shared-variable ".\\RobotBrainExLibrary.lvlib\\WhereAmI? Clean"() -> (w375:T2)  [unwired: 1 in, 1 out]
                      "WhereAmI? Clean" <- w375
                      n160 = Get Date/Time In Seconds "GetMiissionCurrentTime"() -> (seconds since 1Jan1904=w382:timestamp)
                      n161 = call "WhereForebrainPerception.vi"("Where? Midbrain"=w375) -> ("SimPitchRoll"=w370:dbl, "Where? Forebrain"=→"Where? Forebrain":T2, "(xr,yr)"=w378:cluster{"X":dbl, "Y":dbl}, "Direction"=w380:dbl)  [unwired: 3 in]
                      "(xr,yr) A" <- w378
                      n162 = To Double Precision Float(number=w382) -> (double precision float=w383:dbl)
                      n163 = local read "SteerAngle"() -> (w369:dbl)
                      n164 = local read item#-1() -> (w372)
                      n165 = Subtract(x=w383, y=w381) -> (x-y=w384:dbl)
                      n166 = Not(x=w373) -> (.not. x?=w386:bool)
                      n167 = call "DrawRobot.vi"("(xr,yr) old"=w379, "(xr,yr) new"=w378, "2D Picture"=w368) -> ("new picture"=w366:picture)
                      n168 = Divide(x=w384, y=60.0) -> (x/y=w374:dbl)
                      n169 = Select(t=w367, f=w366) -> (s=w377:bool, s? t:f=w365:picture)
                      n170 = shared-variable ".\\RobotBrainExLibrary.lvlib\\MissionTime"(w374) -> ()  [unwired: 1 in, 1 out]
                      n171 = Bundle("Direction"=w380, "SteerAngle"=w369) -> (w371:cluster{"Direction":dbl, "SteerAngle":dbl})  [unwired: 1 in]
                      n172 = Wait (ms)(milliseconds to wait=u32 500) -> ()  [unwired: 1 out]
                    }
                    n173 = while {
                      shift-right: [w358] -> _
                      shift-left: _ -> [w360]
                      stop <- w357 stop-if-true
                      # "WhatIsAroundMe?"
                      n174 = shared-variable ".\\RobotBrainExLibrary.lvlib\\WhatAroundMe? Clean"() -> (w355:cluster{"T":dbl, "Range":dbl, "Bearing":dbl}[])  [unwired: 1 in, 1 out]
                      "What?Midbrain" <- w355
                      n175 = call "WhatForebrainPerception.vi"("What?Midbrain"=w355) -> ("What?Midbrain 2"=→"What?Forebrain":cluster{"T":dbl, "Range":dbl, "Bearing":dbl}[])  [unwired: 2 in]
                      n176 = call "ProcessLidarData.vi"("WhatAroundMe?MM"=w355) -> ("Collision"=w354:bool, "data array [mag, phase (deg)]"=w359:cluster{"magnitude":dbl, "phase":dbl}[])
                      "CollisionLight 2" <- w354
                      n177 = call "SimLIDARPlot.vi"("data array [mag, phase (deg)]"=w359) -> ()  [unwired: 1 in, 1 out]
                      n178 = local read item#-1() -> (w357)
                      n179 = Not(x=w360) -> (.not. x?=w358:bool)
                      n180 = case shown="True" w354 {
                        frame False {
                          # "No \nBeep"
                        }
                        frame True {
                          n181 = call <vilib>:"Beep.vi"("use system alert? (T)"=TRUE, "duration (msec)"=u32 1000, "frequency (Hz)"=u32 900) -> ()  [unwired: 9 in]
                        }
                      }
                      n182 = Wait (ms)(milliseconds to wait=u32 100) -> ()  [unwired: 1 out]
                    }
                    n183 = disable-structure shown="Disabled" {
                      frame Disabled {
                        n184 = while {
                          shift-right: [w333] -> _
                          shift-left: _ -> [w332]
                          shift-right: [w325] -> _
                          shift-left: 0.0 ("SteerAngle") -> [w324]
                          stop <- w335 stop-if-true
                          # "Neo-Cortex"
                          n185 = local read item#-1() -> (w317)
                          n186 = local read "MDF"() -> (w316:T6)
                          n187 = Not(x=w332) -> (.not. x?=w333:bool)
                          n188 = Not() -> (.not. x?=w321:bool)  [unwired: 1 in]
                          n189 = Select(t=w317, f=w316) -> (s=w315:bool, s? t:f=w314:T6)
                          n190 = Or(x=w321, y="E-Stop") -> (x .or. y?=w319:bool)
                          n191 = Not(x=w319) -> (.not. x?=w318:bool)
                          n192 = local read item#-1() -> (w335)
                          n193 = local read "Where? Forebrain"() -> (w331:T2)
                          n194 = local read "What?Forebrain"() -> (w330:cluster{"T":dbl, "Range":dbl, "Bearing":dbl}[])
                          n195 = Boolean To (0,1)(Boolean=w318) -> (0, 1=w323:i16)
                          n196 = To Double Precision Float(number=w323) -> (double precision float=w322:dbl)
                          n197 = call "GotoWaypoint.vi"("SupressIn"=w322, "InhibitIn"=FALSE, "CurrentSteerAngle"=w324, "WhatAroundMe? Clean"=w330, "WhereAmI? Clean"=w331, "MDF In"=w314) -> ("MDF Out"=w327:T6, "ActCommand"=→"NeoActCom":dbl[], "Vel"=w326:dbl, "SteerAngle"=w325:dbl)  [unwired: 2 out]
                          "SteerAngle" <- w325
                          "MDF Out" <- w327
                          n198 = local write "MDF"(w327) -> ()
                          n199 = Wait (ms)(milliseconds to wait=u32 100) -> ()  [unwired: 1 out]
                        }
                      }
                      frame Enabled {
                      }
                    }
                    n200 = while {
                      shift-right: [w352] -> _
                      shift-left: _ -> [w348]
                      stop <- w347 stop-if-true
                      # "HowAmI?"
                      n201 = shared-variable ".\\RobotBrainExLibrary.lvlib\\HowAmI? Clean"() -> (w349:cluster{"T":dbl, "Battery":dbl, "Temp":dbl})  [unwired: 1 in, 1 out]
                      "How?Midbrain" <- w349
                      n202 = call "HowForebrainPerception.vi"("How?MidbrainIn"=w349) -> (2:w350, 3:→"How?Forebrain")  [unwired: 1 in, 1 out]
                      n203 = local read item#-1() -> (w347)
                      n204 = Not(x=w348) -> (.not. x?=w352:bool)
                      n205 = Wait (ms)(milliseconds to wait=u32 1000) -> ()  [unwired: 1 out]
                    }
                    n206 = while {
                      shift-right: [w337] -> _
                      shift-left: _ -> [w338]
                      stop <- w340 stop-if-true
                      # "HypoThallumus"
                      n207 = Not(x=w338) -> (.not. x?=w337:bool)
                      n208 = call "Hypo-T.vi"() -> ("Hypo T Act Out"=→"Hypo Out":cluster{"Motor1":i16, "Motor 2":i16})  [unwired: 3 in]
                      n209 = local read item#-1() -> (w340)
                      n210 = Wait (ms)(milliseconds to wait=u32 800) -> ()  [unwired: 1 out]
                    }
                    n211 = while {
                      shift-right: [w345] -> _
                      shift-left: _ -> [w344]
                      stop <- w343 stop-if-true
                      # "ForebrainAct"
                      n212 = local read "NeoActCom"() -> (w342:dbl[])
                      n213 = local read item#-1() -> (w343)
                      n214 = Not(x=w344) -> (.not. x?=w345:bool)
                      n215 = call "ForebrainArbiter.vi"(0:w342) -> ("ForebrainActCom"=w341:dbl[])  [unwired: 14 in]
                      n216 = shared-variable ".\\RobotBrainExLibrary.lvlib\\ActCommand"(w341) -> ()  [unwired: 1 in, 1 out]
                      n217 = Wait (ms)(milliseconds to wait=u32 100) -> ()  [unwired: 1 out]
                    }
                  }
                  frame #2 {
                    (unwired) T19 {"VelCom"=0.0, "BehCom"=enum."OpenFieldTransit"} ("ForebrainCom")
                    w392 = T18."Startup&Shutdown" ("Tab")
                    # "Set robot Vel to 0"
                    # "Reset latched run\nswitch"
                    # "Force control to\nShutdown Case"
                    n218 = local write "Main Tab Interface"(w392) -> ()
                    n219 = Initialize Array(0.0 ("element"), 90 ("dimension size")) -> (w388:dbl[])
                    n220 = shared-variable ".\\RobotBrainExLibrary.lvlib\\ActCommand"(w388) -> ()  [unwired: 1 in, 1 out]
                    n221 = local write item#-1(TRUE ("RunAutoMode")) -> ()
                  }
                }
              }
              frame Enabled {
              }
            }
          }
          frame 7 {
            n222 = Wait (ms)(milliseconds to wait=u32 500) -> ()  [unwired: 1 out]
          }
          frame 2 {
            w402 = T18."Startup&Shutdown" ("Tab")
            # "Put code here in place of delay"
            # "Sends Tab Control\nback to Startup\ncase"
            n223 = Wait (ms)(milliseconds to wait=u32 2000) -> ()  [unwired: 1 out]
            n224 = local write "Main Tab Interface"(w402) -> ()
          }
        }
        n225 = Not(x=w47) -> (.not. x?=w30:bool)
        "Robot Live" <- w30
      }
    }
    frame #2 {
      # "Realease LIDAR\nMemory"
      # "Reset Run \nSwitch"
      # "Shutdown Robot"
      n226 = call "Pixel_LIDAR_Close.vi"("error in (no error) 2"=w404, "Image"=w405) -> ()  [unwired: 1 in]
      n227 = local write "RunRobot"(TRUE ("RunRobot")) -> ()
    }
  }
